vi "SPI.vi"(11 "data":u32) -> ()   [LabVIEW 2015]
uses:
  <vilib>/DAQmx/write.llb/DAQmx Write (Digital Bool 1Line 1Point).vi
  <vilib>/DAQmx/create/channels.llb/DAQmx Create Channel (DO-Digital Output).vi
  data.vi
  <vilib>/DAQmx/miscellaneous.llb/DAQmx Fill In Error Info.vi
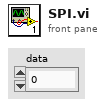
[diagram p1: front panel]
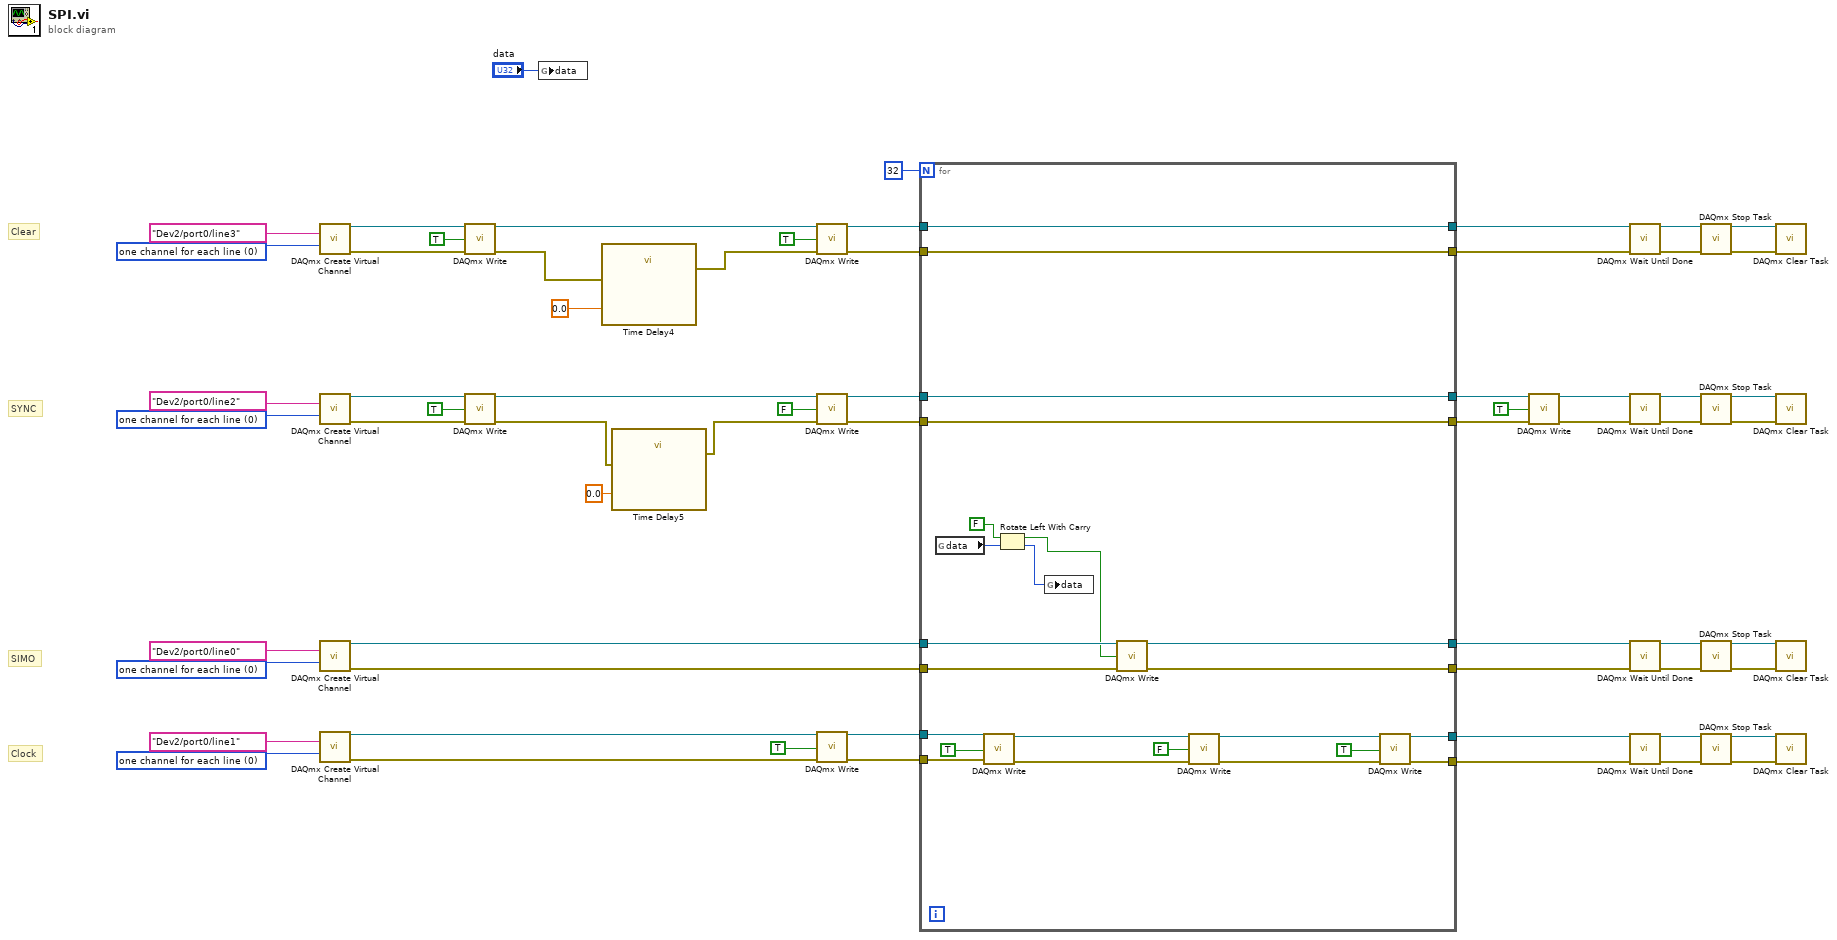
[diagram p0: block diagram]
diagram:
  w41 = 0 items=["one channel for each line", "one channel for all lines"] ("line grouping")
  w44 = 0 items=["one channel for each line", "one channel for all lines"] ("line grouping")
  w60 = 0 items=["one channel for each line", "one channel for all lines"] ("line grouping")
  w62 = 0 items=["one channel for each line", "one channel for all lines"] ("line grouping")
  # "SYNC"
  # "Clock"
  # "SIMO"
  # "Clear"
  n1 = call-poly <vilib>:"DAQmx Create Virtual Channel.vi"("lines"=tag "Dev2/port0/line3", "line grouping"=w41) -> ("task out"=w39:refnum<k21>, "error out"=w38:errorcluster)  [unwired: 12 in]
  n2 = call-poly <vilib>:"DAQmx Create Virtual Channel.vi"("lines"=tag "Dev2/port0/line2", "line grouping"=w44) -> ("task out"=w24:refnum<k21>, "error out"=w23:errorcluster)  [unwired: 12 in]
  n3 = call-poly <vilib>:"DAQmx Create Virtual Channel.vi"("lines"=tag "Dev2/port0/line0", "line grouping"=w62) -> ("task out"=w51:refnum<k21>, "error out"=w52:errorcluster)  [unwired: 12 in]
  n4 = call-poly <vilib>:"DAQmx Create Virtual Channel.vi"("lines"=tag "Dev2/port0/line1", "line grouping"=w60) -> ("task out"=w4:refnum<k21>, "error out"=w3:errorcluster)  [unwired: 12 in]
  n5 = call-poly <vilib>:"DAQmx Write.vi"("task/channels in"=w39, "data"=TRUE, "error in"=w38) -> ("task out"=w34:refnum<k21>, "error out"=w36:errorcluster)  [unwired: 10 in, 1 out]
  n6 = call-poly <vilib>:"DAQmx Write.vi"("task/channels in"=w24, "data"=TRUE, "error in"=w23) -> ("task out"=w21:refnum<k21>, "error out"=w22:errorcluster)  [unwired: 10 in, 1 out]
  n7 = global write "data.vi" "data"("data") -> ()
  n8 = call "Time Delay4"("error in (no error)"=w36, "Delay Time (s)"=0.0) -> ("error out"=w33:errorcluster)  [unwired: 9 in]
  n9 = call "Time Delay5"("error in (no error)"=w22, "Delay Time (s)"=0.0) -> ("error out"=w31:errorcluster)  [unwired: 9 in]
  n10 = call-poly <vilib>:"DAQmx Write.vi"("task/channels in"=w34, "data"=TRUE, "error in"=w33) -> ("task out"=w8:refnum<k21>, "error out"=w6:errorcluster)  [unwired: 10 in, 1 out]
  n11 = call-poly <vilib>:"DAQmx Write.vi"("task/channels in"=w21, "data"=FALSE, "error in"=w31) -> ("task out"=w28:refnum<k21>, "error out"=w26:errorcluster)  [unwired: 10 in, 1 out]
  n12 = call-poly <vilib>:"DAQmx Write.vi"("task/channels in"=w4, "data"=TRUE, "error in"=w3) -> ("task out"=w1:refnum<k21>, "error out"=w2:errorcluster)  [unwired: 10 in, 1 out]
  n13 = for {
    N: 32 -> [_]
    tunnel: w52 -> [w71]
    tunnel: w51 -> [w86]
    tunnel: [w85] -> w50
    tunnel: [w84] -> w49
    tunnel: w1 -> [w83]
    tunnel: [w65] -> w48
    tunnel: [w66] -> w47
    tunnel: w2 -> [w81]
    tunnel: [w75] -> w29
    tunnel: w28 -> [w75]
    tunnel: [w74] -> w27
    tunnel: w26 -> [w74]
    tunnel: [w73] -> w9
    tunnel: w8 -> [w73]
    tunnel: [w72] -> w7
    tunnel: w6 -> [w72]
    n14 = global read "data.vi" "data"() -> (w79:u32)
    n15 = call-poly <vilib>:"DAQmx Write.vi"("task/channels in"=w83, "data"=TRUE, "error in"=w81) -> ("task out"=w82:refnum<k21>, "error out"=w70:errorcluster)  [unwired: 10 in, 1 out]
    n16 = Rotate Left With Carry(2:w79, 3:FALSE ("carry")) -> (0:w78:u32, 1:w76:bool)
    n17 = global write "data.vi" "data"(w78) -> ()
    n18 = call-poly <vilib>:"DAQmx Write.vi"("task/channels in"=w86, "data"=w76, "error in"=w71) -> ("task out"=w85:refnum<k21>, "error out"=w84:errorcluster)  [unwired: 10 in, 1 out]
    n19 = call-poly <vilib>:"DAQmx Write.vi"("task/channels in"=w82, "data"=FALSE, "error in"=w70) -> ("task out"=w68:refnum<k21>, "error out"=w67:errorcluster)  [unwired: 10 in, 1 out]
    n20 = call-poly <vilib>:"DAQmx Write.vi"("task/channels in"=w68, "data"=TRUE, "error in"=w67) -> ("task out"=w65:refnum<k21>, "error out"=w66:errorcluster)  [unwired: 10 in, 1 out]
  }
  n21 = call-poly <vilib>:"DAQmx Write.vi"("task/channels in"=w29, "data"=TRUE, "error in"=w27) -> ("task out"=w15:refnum<k21>, "error out"=w14:errorcluster)  [unwired: 10 in, 1 out]
  n22 = call <vilib>:"DAQmx Wait Until Done.vi"("task/channels in"=w9, "error in"=w7) -> ("task out"=w11:refnum<k21>, "error out"=w10:errorcluster)  [unwired: 12 in]
  n23 = call <vilib>:"DAQmx Wait Until Done.vi"("task/channels in"=w15, "error in"=w14) -> ("task out"=w17:refnum<k21>, "error out"=w16:errorcluster)  [unwired: 12 in]
  n24 = call <vilib>:"DAQmx Wait Until Done.vi"("task/channels in"=w50, "error in"=w49) -> ("task out"=w56:refnum<k21>, "error out"=w55:errorcluster)  [unwired: 12 in]
  n25 = call <vilib>:"DAQmx Wait Until Done.vi"("task/channels in"=w48, "error in"=w47) -> ("task out"=w54:refnum<k21>, "error out"=w53:errorcluster)  [unwired: 12 in]
  n26 = call <vilib>:"DAQmx Stop Task.vi"("task/channels in"=w11, "error in"=w10) -> ("task out"=w13:refnum<k21>, "error out"=w12:errorcluster)  [unwired: 12 in]
  n27 = call <vilib>:"DAQmx Stop Task.vi"("task/channels in"=w17, "error in"=w16) -> ("task out"=w19:refnum<k21>, "error out"=w18:errorcluster)  [unwired: 12 in]
  n28 = call <vilib>:"DAQmx Stop Task.vi"("task/channels in"=w56, "error in"=w55) -> ("task out"=w64:refnum<k21>, "error out"=w63:errorcluster)  [unwired: 12 in]
  n29 = call <vilib>:"DAQmx Stop Task.vi"("task/channels in"=w54, "error in"=w53) -> ("task out"=w58:refnum<k21>, "error out"=w57:errorcluster)  [unwired: 12 in]
  n30 = call <vilib>:"DAQmx Clear Task.vi"("task in"=w13, "error in"=w12) -> ()  [unwired: 13 in, 1 out]
  n31 = call <vilib>:"DAQmx Clear Task.vi"("task in"=w19, "error in"=w18) -> ()  [unwired: 13 in, 1 out]
  n32 = call <vilib>:"DAQmx Clear Task.vi"("task in"=w64, "error in"=w63) -> ()  [unwired: 13 in, 1 out]
  n33 = call <vilib>:"DAQmx Clear Task.vi"("task in"=w58, "error in"=w57) -> ()  [unwired: 13 in, 1 out]
